vi "for_condicional.vi"() -> ()   [LabVIEW 2020]
panel:
  out "Array 3":dbl[](array[numeric])
  out "Array 2":i32[](array[numeric])
  out "Array":i32[](array[numeric])
  out "numero \nde iteracion":i32
  # "for"
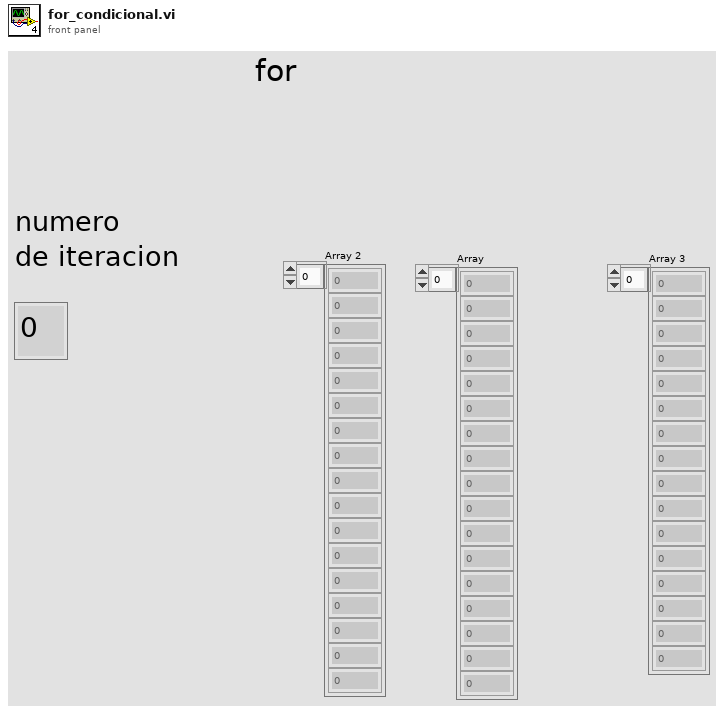
[diagram p1: front panel]
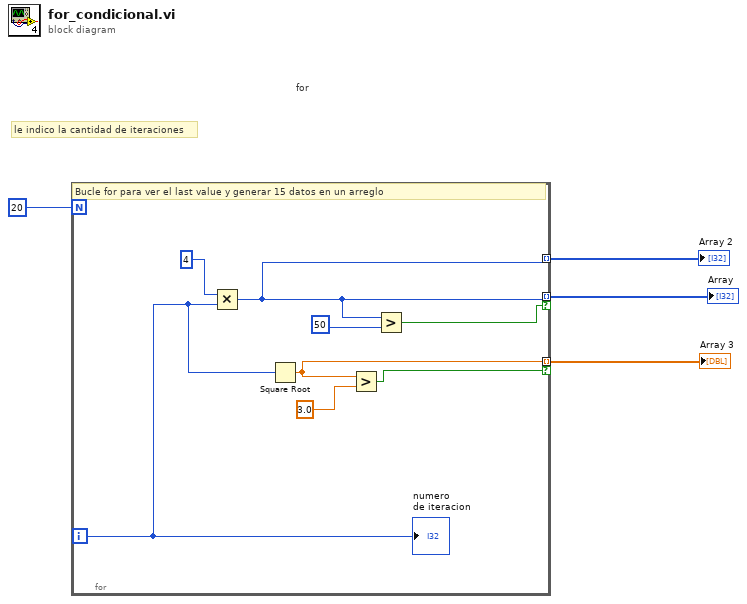
[diagram p0: block diagram]
diagram:
  # "le indico la cantidad de iteraciones"
  # "for"
  n1 = for {
    N: 20 -> [_]
    tunnel: [w9] -> w3 mode=indexing if=w10
    tunnel: [w9] -> w2 mode=indexing
    tunnel: [w6] -> w1 mode=indexing if=w5
    i -> [w8]
    # "Bucle for para ver el last value y generar 15 datos en un arreglo"
    n2 = Multiply(x=4, y=w8) -> (x*y=w9:i32)
    n3 = Square Root(x=w8) -> (sqrt(x)=w6:dbl)
    n4 = Greater?(x=w6, y=3.0) -> (0:w5:bool)
    n5 = Greater?(x=w9, y=50) -> (0:w10:bool)
    "numero \nde iteracion" <- w8
  }
  "Array" <- w3
  "Array 2" <- w2
  "Array 3" <- w1
